vi "LoadApp.vi"(8 "error in (no error)":errorcluster, 11 "arguments":string[](array[string])) -> (0 "error out":errorcluster)   [LabVIEW 2019, in "TestBench.lvlib" / "TestBench.lvclass"]
uses:
  TestBench/TestBench.lvclass
  C:/Program Files (x86)/National Instruments/LabVIEW 2019/vi.lib/ActorFramework/Actor/Actor.lvclass
  <vilib>/ActorFramework/Actor/Actor.lvclass
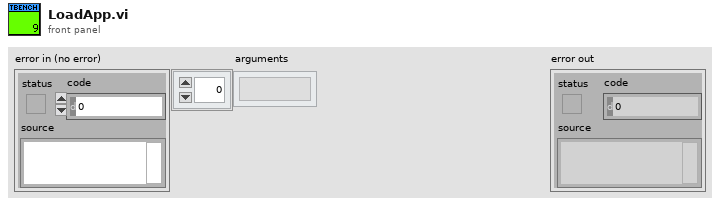
[diagram p1: front panel]
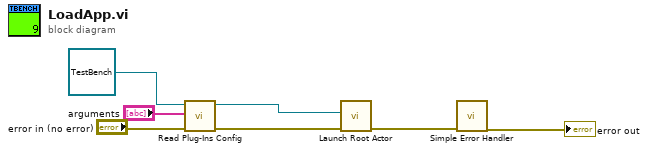
[diagram p0: block diagram]
diagram:
  n1 = call-dynamic "Read Plug-Ins Config.vi"("error in (no error)"="error in (no error)", "arguments"="arguments", "TestBench in"=refnum<class "TestBench.lvclass"> refnum ("TestBench.lvlib:TestBench.lvclass")) -> ("error out"=w3:errorcluster, "TestBench out"=w5:refnum<class "TestBench.lvclass">)  [unwired: 7 in]
  n2 = call <vilib>:"Launch Root Actor.vi"("error in (no error)"=w3, "Actor"=w5) -> ("error out"=w7:errorcluster)  [unwired: 8 in, 1 out]
  n3 = call <vilib>:"Simple Error Handler.vi"("error in (no error)"=w7) -> ("error out"=→"error out":errorcluster)  [unwired: 4 in, 4 out]
